vi "Call Defragment.vi"(8 "error in":errorcluster, 11 "TDMS in":refnum<class "TDMS.lvclass">) -> (0 "error out":errorcluster, 3 "TDMS out":refnum<class "TDMS.lvclass">)   [LabVIEW 2019, in "TDMS.lvlib" / "TDMS.lvclass"]
uses:
  TDMS.lvclass
  C:/Users/Public/Documents/Development/builds/Tools/Report.lvlibp/Report.lvclass
  Defragment.vi
  builds/Tools/Report.lvlibp/Accessors/Read Root Path.vi
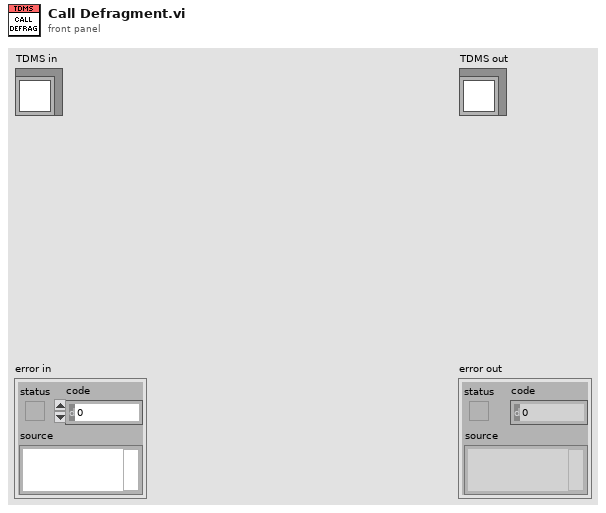
[diagram p1: front panel]
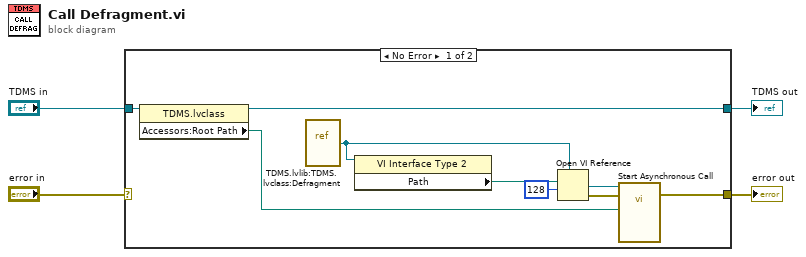
[diagram p0: block diagram]
diagram:
  n1 = case shown="No Error" "error in" {
    selector: "error in" -> [_ w15]
    tunnel: [w5 w15] -> w3
    tunnel: [w7 w14] -> w1
    tunnel: "TDMS in" -> [w8 w14]
    frame No Error {
      n2 = property class="TDMS.lvclass"(reference=w8) -> (reference out=w7:refnum<class "TDMS.lvclass">, "Accessors:Root Path"=w6:path)  [unwired: 1 in, 1 out]
      n3 = vi-ref "TDMS.lvlib:TDMS.lvclass:Defragment.vi"() -> (w11:refnum<vi>)
      n4 = property class="VI Interface Type 2"(reference=w11) -> ("Path"=w9:path)  [unwired: 1 in, 2 out]
      n5 = Open VI Reference(type specifier VI Refnum (for type only)=w11, vi path=w9, options=128) -> (vi reference=w12:refnum<vi>, error out=w13:errorcluster)  [unwired: 3 in]
      n6 = call-by-ref "Start Asynchronous Call"(reference=w12, error in=w13, "Path"=w6) -> (error out=w5:errorcluster)  [unwired: 10 in, 2 out]
    }
    frame Error {
    }
  }
  "error out" <- w3
  "TDMS out" <- w1
